vi "Write ITX.vi"(6 "Commands":string, 8 "error in":errorcluster, 9 "Notes":string, 10 "Data (Dictionary)":T1[](array[typedef]), 11 "filename":path) -> (0 "error out":errorcluster, 3 "file":path)   [LabVIEW 2019, in "Data.ITX.lvclass"]
uses:
  Data.ITX.lvclass
  <vilib>/addons/_JKI.lib/Serialization/JSON/Serializer/JSON Serializer/JSON Serializer.lvclass
  Data/Typedefs/Dictionary--cluster.ctl
  Data/Data.lvclass
panel:
  out "String":string
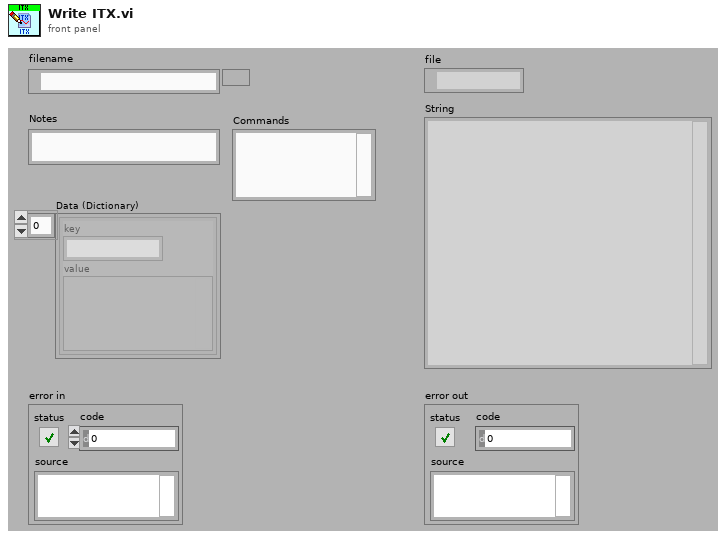
[diagram p1: front panel]
types:
  T1 = typedef "Data.lvclass/Dictionary--cluster.ctl" = cluster{"key":string, "value":variant}
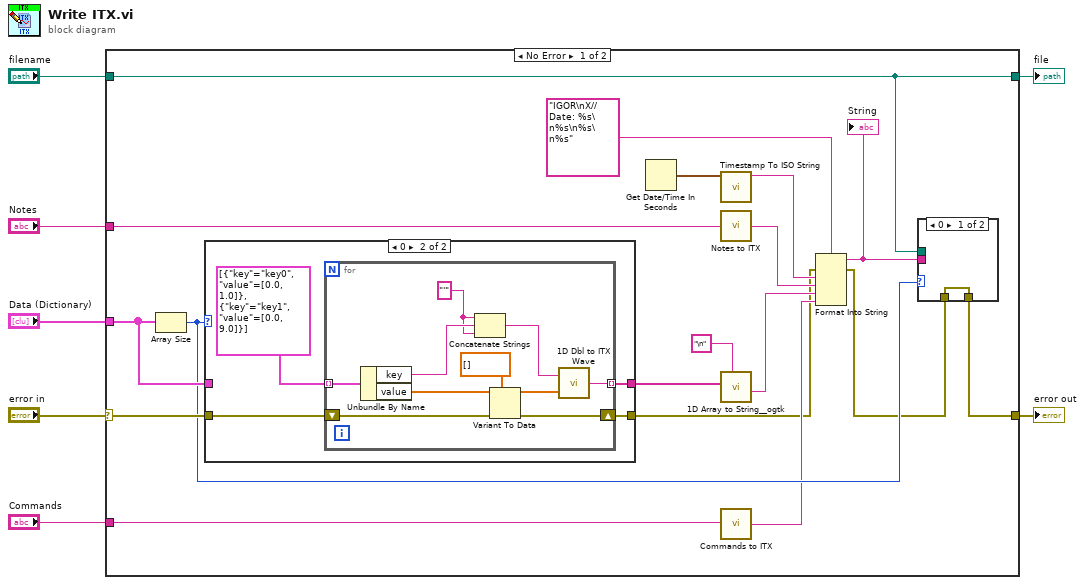
[diagram p0: block diagram]
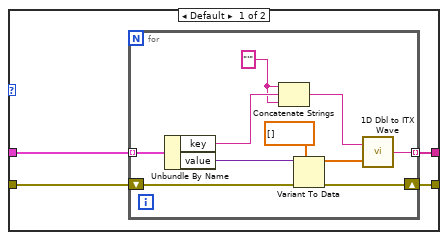
[diagram p2: hidden frame]
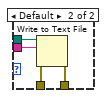
[diagram p3: hidden frame]
diagram:
  n1 = case shown="No Error" "error in" {
    selector: "error in" -> [w21 w59]
    tunnel: "filename" -> [w22 w60]
    tunnel: "Notes" -> [w25 _]
    tunnel: [w24 w59] -> w5
    tunnel: "Data (Dictionary)" -> [w23 _]
    tunnel: [w22 w60] -> w3
    tunnel: "Commands" -> [w20 _]
    frame No Error {
      n2 = Array Size(array=w23) -> (size(s)=w18:i32)
      n3 = case shown="0" w18 {
        tunnel: [w29 w43] -> w19
        tunnel: w23 -> [w28 _]
        tunnel: w21 -> [w27 w42]
        tunnel: [w26 w41] -> w10
        frame Default {
          n4 = for {
            tunnel: [w39] -> w29 mode=indexing
            tunnel: w28 -> [w37] mode=indexing
            shift-right: [w32] -> w26
            shift-left: w27 -> [w33]
            w30 = "'"
            n5 = Unbundle By Name(w37) -> ("key"=w31:string, "value"=w35:variant)
            n6 = Concatenate Strings(w30, w31, w30) -> (w38:string)
            n7 = Variant To Data(error in=w33, type=dbl[] [] ("Data"), Variant=w35) -> (data=w34:dbl[], error out=w32:errorcluster)
            n8 = call "1D Dbl to ITX Wave.vi"("1D Array"=w34, "Wavename"=w38) -> ("ITX Wave"=w39:string)
          }
        }
        frame 0 {
          n9 = for {
            tunnel: [w53] -> w43 mode=indexing
            tunnel: cluster{"key":string, "value":dbl[]}[] [{"key"="key0", "value"=[0.0, 1.0]}, {"key"="key1", "value"=[0.0, 9.0]}] ("Data (Dictionary)") -> [w51] mode=indexing
            shift-right: [w46] -> w41
            shift-left: w42 -> [w47]
            w44 = "'"
            n10 = Unbundle By Name(w51) -> ("key"=w45:string, "value"=w49:dbl[])
            n11 = Concatenate Strings(w44, w45, w44) -> (w52:string)
            n12 = Variant To Data(error in=w47, type=dbl[] [] ("Data"), Variant=w49) -> (data=w48:dbl[], error out=w46:errorcluster)
            n13 = call "1D Dbl to ITX Wave.vi"("1D Array"=w48, "Wavename"=w52) -> ("ITX Wave"=w53:string)
          }
        }
      }
      n14 = Get Date/Time In Seconds() -> (seconds since 1Jan1904=w13:timestamp)
      n15 = call <vilib>:"Timestamp To ISO String.vi"("Timestamp"=w13) -> ("ISO Timestamp String"=w12:string)  [unwired: 9 in, 1 out]
      n16 = call "Notes to ITX.vi"("Notes"=w25) -> ("ITX Notes"=w17:string)
      n17 = call "1D Array to String__ogtk.vi"("delimiter (Tab)"="\n", "Array of Strings"=w19) -> ("delimited string"=w16:string)  [unwired: 9 in]
      n18 = call "Commands to ITX.vi"("Commands"=w20) -> ("ITX Commands"=w15:string)
      n19 = Format Into String(format string="IGOR\nX// Date: %s\n%s\n%s\n%s", error in=w10, w12, w17, w16, w15) -> (resulting string=w8:string, error out=w9:errorcluster)  [unwired: 1 in]
      "String" <- w8
      n20 = case shown="0" w18 {
        tunnel: w8 -> [_ w58]
        tunnel: [w54 w57] -> w24
        tunnel: w9 -> [w54 w56]
        tunnel: w22 -> [_ w55]
        frame 0 {
        }
        frame Default {
          n21 = Write to Text File(file (use dialog)=w55, text=w58, error in=w56) -> (error out=w57:errorcluster)  [unwired: 3 out]
        }
      }
    }
    frame Error {
    }
  }
  "file" <- w3
  "error out" <- w5
